vi "ExWrite1File.vi"() -> ()   [LabVIEW 2010]
panel:
  out "Hidden File Type":i32
  out "error out":errorcluster
  in  "error in (no error)":errorcluster
  out "?":string
  in  "?":bool
  in  "Y Size":u32=1 min=1 step=1
  in  "X Size":u32=1 min=1 step=1
  in  "File Name":path
  in  "Data Type":u16(ring)=1 items=["8 Bit Unsigned Integer", "16 Bit Unsigned Integer", "32 Bit Unsigned Integer", "32 Bit Floating Point"]
  in  "File Type":u16(ring)=1 items=["PMI (Photometrics)", "SPE (Princeton Instruments)", "TIFF"]
  # "ExWriteOneFile.vi\nThis Example will create a new file of the type specified\nand fill it with demo data of the form p(x,y) = (y*100) + x.\nIt uses an event loop to set the file type in the brower\nas it is selected."
  # "NOTICE\n\nTHIS VI REQUIRES THAT THE TOOLKIT\nBE UNLOADED BY RUNNING THE\n VI EXCLOSEGLOBALCAM.VI\n BEFORE LEAVING LABVIEW."
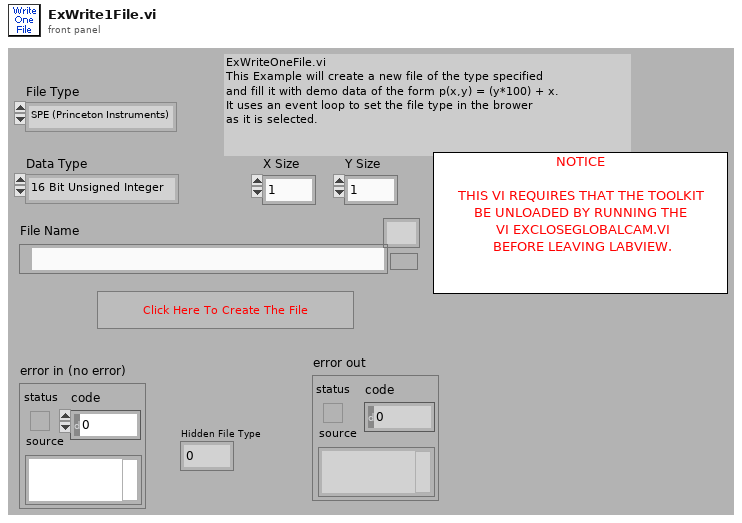
[diagram p1: front panel]
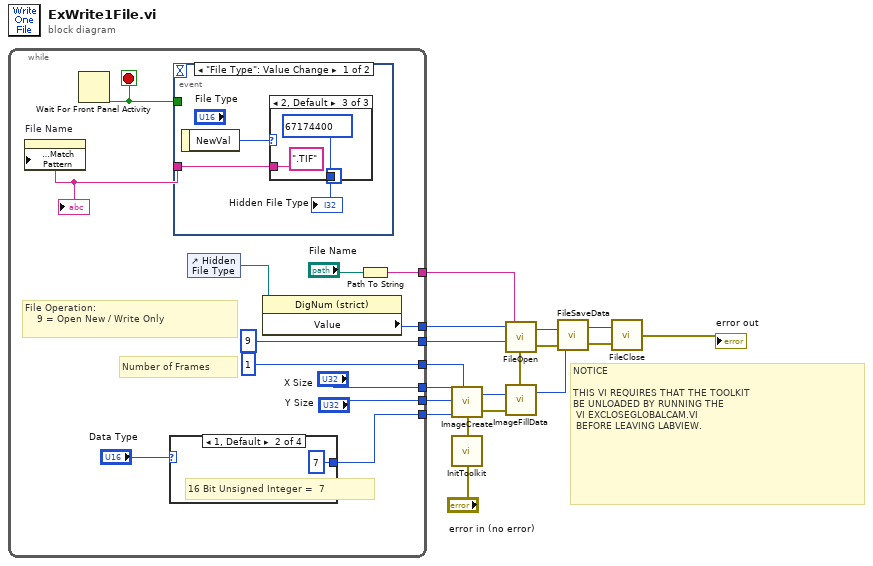
[diagram p0: block diagram]
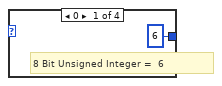
[diagram p2: hidden frame]
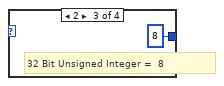
[diagram p3: hidden frame]
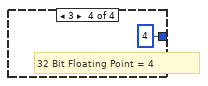
[diagram p4: hidden frame]
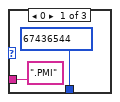
[diagram p5: hidden frame]
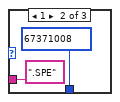
[diagram p6: hidden frame]
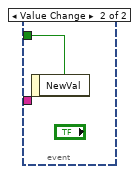
[diagram p7: hidden frame]
diagram:
  # "NOTICE\n\nTHIS VI REQUIRES THAT THE TOOLKIT\nBE UNLOADED BY RUNNING THE\n VI EXCLOSEGLOBALCAM.VI\n BEFORE LEAVING LABVIEW."
  n1 = while {
    tunnel: [1] -> w16
    tunnel: ["X Size"] -> w12
    tunnel: ["Y Size"] -> w11
    tunnel: [w27] -> w10
    tunnel: [9] -> w9
    tunnel: [w19] -> w4
    tunnel: [w21] -> w2
    stop <- w24 stop-if-true
    # "Number of Frames"
    # "File Operation:\n    9 = Open New / Write Only"
    n2 = case shown="1, Default" "Data Type" {
      tunnel: [6 7 8 4] -> w19
      frame 0 {
        # "8 Bit Unsigned Integer =  6"
      }
      frame 1, Default {
        # "16 Bit Unsigned Integer =  7"
      }
      frame 2 {
        # "32 Bit Unsigned Integer =  8"
      }
      frame 3 {
        # "32 Bit Floating Point = 4"
      }
    }
    n3 = event shown="[0] \"File Type\": Value Change" {
      selector: _ -> [_ _]
      dyn-events: _ -> [_ _]
      timeout: _ -> [_ _]
      tunnel: [w36 _] -> w23
      tunnel: [_ w44] -> w24
      event "File Type": Value Change {
        n4 = event-data() -> ("NewVal"=w37:u16)  [unwired: 1 in]
        n5 = case shown="2, Default" w37 {
          tunnel: [67436544 67371008 67174400] -> w35
          tunnel: [".PMI" ("String") ".SPE" ("String") ".TIF" ("String")] -> w36
          frame 0 {
          }
          frame 1 {
          }
          frame 2, Default {
          }
        }
        "Hidden File Type" <- w35
      }
      event Value Change {
        n6 = event-data() -> ("NewVal"=w44:bool)  [unwired: 1 in]
      }
    }
    "?" <- w23
    n7 = property on="File Name" class="Path"("Browse Options:Match Pattern"=w23) -> ()  [unwired: 2 in, 2 out]
    n8 = Wait For Front Panel Activity(3:w24) -> ()  [unwired: 2 in, 1 out]
    n9 = control-ref of="Hidden File Type"() -> (w22:refnum<vi>)
    n10 = property class="DigNum (strict)"(reference=w22) -> ("Value"=w21:i32)  [unwired: 1 in, 2 out]
    n11 = Path To String(path="File Name") -> (string=w27:string)
  }
  n12 = call <userlib>:"InitToolkit.vi"("error in"="error in (no error)") -> ("error out"=w5:errorcluster)
  n13 = call <userlib>:"ImageCreate.vi"("X dimension"=w12, "Y dimension"=w11, "Data Type"=w4, "error in"=w5, "Number Of Frames"=w16) -> ("Image Handle"=w17:u32, "error out"=w18:errorcluster)
  n14 = call <userlib>:"ImageFillData.vi"("error in"=w18, "Image Handle"=w17) -> ("error out"=w8:errorcluster, "Image Handle"=w14:u32)  [unwired: 1 in]
  n15 = call <userlib>:"FileOpen.vi"("error in"=w8, "File Operations"=w9, "FileName"=w10, "File Type"=w2) -> ("error out"=w7:errorcluster, "File Handle"=w6:u32)
  n16 = call <userlib>:"FileSaveData.vi"("error in"=w7, "Image Handle"=w14, "File Handle"=w6) -> ("error out"=w15:errorcluster, "File Handle"=w13:u32)
  n17 = call <userlib>:"FileClose.vi"("error in"=w15, "File Handle"=w13) -> ("error out"=→"error out":errorcluster)
